vi "WavaFrequencyMeasurement.vi"() -> ()   [LabVIEW 2019]
uses:
  <vilib>/rvi/Emulation/niFpgaGetClockAttributes.vi
  <vilib>/rvi/Emulation/niFpgaSctlEmulationGetInTimedLoop.vi
  <vilib>/rvi/Emulation/niFpgaEmulationReportErrorSimple.vi
  <vilib>/rvi/eio/common/nirviEmuTemplateMethod_errors.vi
  <vilib>/rvi/Emulation/niFpgaCriticalErrorInLSC.vi
  <vilib>/eio/EIONode/EIONode.xnode
panel:
  out "数值":u32
  out "x+1":u32
  out "被测信号个数":u32
  out "时钟信号个数":u32
  in  "Count(Ticks)":u32=8 caption="计数器(滴答)"
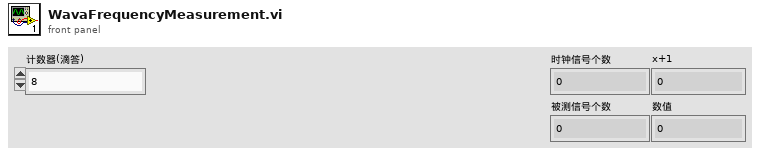
[diagram p1: front panel]
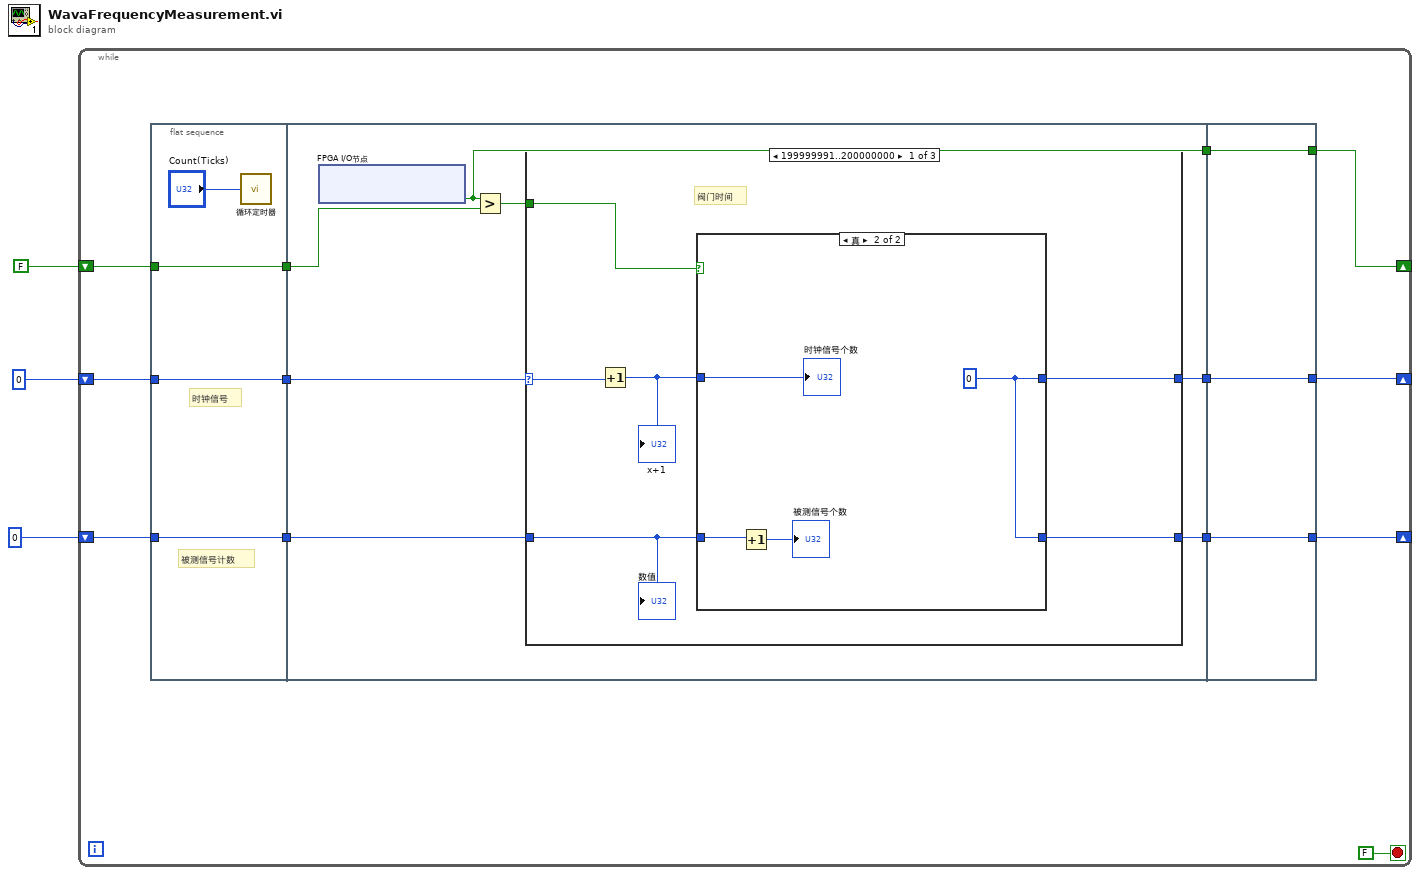
[diagram p0: block diagram]
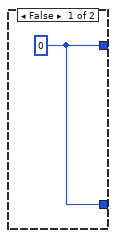
[diagram p2: hidden frame]
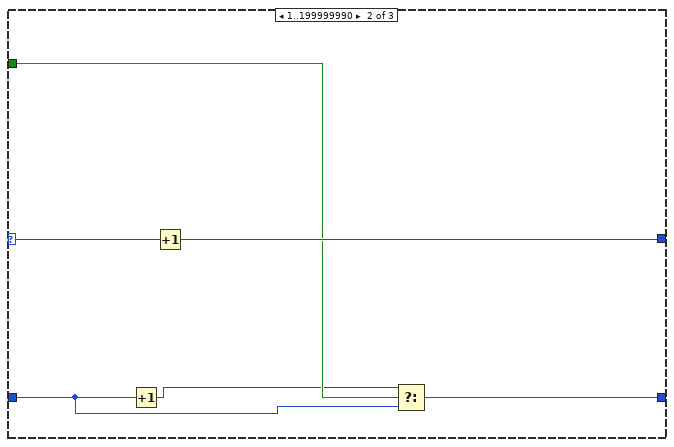
[diagram p3: hidden frame]
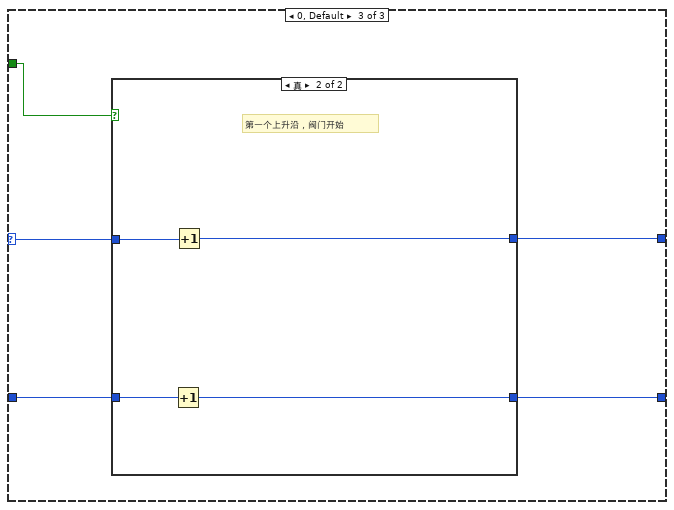
[diagram p4: hidden frame]
diagram:
  n1 = while {
    shift-right: [w7] -> _
    shift-left: FALSE -> [w14]
    shift-right: [w9] -> _
    shift-left: u32 0 -> [w12]
    shift-right: [w8] -> _
    shift-left: u32 0 -> [w10]
    stop <- FALSE stop-if-true
    n2 = flat-sequence {
      tunnel: [w19] -> w15
      tunnel: w14 -> [w19]
      tunnel: [w18] -> w13
      tunnel: w12 -> [w18]
      tunnel: [w17] -> w11
      tunnel: w10 -> [w17]
      tunnel: w15 -> [w27]
      tunnel: w13 -> [w26]
      tunnel: w11 -> [w24]
      tunnel: [w23] -> w6
      tunnel: [w22] -> w5
      tunnel: [w21] -> w4
      tunnel: [w56] -> w7
      tunnel: [w57] -> w8
      tunnel: [w58] -> w9
      tunnel: w6 -> [w58]
      tunnel: w5 -> [w57]
      tunnel: w4 -> [w56]
      frame #0 {
        # "被测信号计数"
        # "时钟信号"
        n3 = call "循环定时器"("Count(Ticks)"="Count(Ticks)") -> ()  [unwired: 1 out]
      }
      frame #1 {
        n4 = xnode "FPGA I/O节点"() -> ("ConnectorB/DIO0"=w21:bool)  [unwired: 1 in, 1 out]
        n5 = Greater?(x=w21, y=w27) -> (0:w25:bool)
        n6 = case "条件结构" shown="199999991..200000000" w26 {
          selector: w26 -> [w32 w44 w48]
          tunnel: w25 -> [w33 w42 w49]
          tunnel: w24 -> [w31 w40 w47]
          tunnel: [w30 w43 w46] -> w23
          tunnel: [w29 w39 w45] -> w22
          frame 199999991..200000000 {
            # "阀门时间"
            n7 = Increment(x=w32) -> (x+1=w28:u32)
            "x+1" <- w28
            n8 = case shown="真" w33 {
              tunnel: w31 -> [_ w37]
              tunnel: [w34 w38] -> w30
              tunnel: [w34 w38] -> w29
              tunnel: w28 -> [_ w35]
              frame False {
                w34 = u32 0
              }
              frame True {
                w38 = u32 0
                n9 = Increment(x=w37) -> (x+1=→"被测信号个数":u32)
                "时钟信号个数" <- w35
              }
            }
            "数值" <- w31
          }
          frame 1..199999990 {
            n10 = Increment(x=w40) -> (x+1=w41:u32)
            n11 = Increment(x=w44) -> (x+1=w43:u32)
            n12 = Select(t=w41, s=w42, f=w40) -> (s? t:f=w39:u32)
          }
          frame 0, Default {
            n13 = case shown="真" w49 {
              tunnel: w48 -> [w51 w55]
              tunnel: w47 -> [w50 w54]
              tunnel: [w51 w53] -> w46
              tunnel: [w50 w52] -> w45
              frame False {
                # "不开始"
              }
              frame True {
                # "第一个上升沿，阀门开始"
                n14 = Increment(x=w54) -> (x+1=w52:u32)
                n15 = Increment(x=w55) -> (x+1=w53:u32)
              }
            }
          }
        }
      }
      frame #2 {
      }
    }
  }
